vi "WriteTree.vi"(8 "error in":errorcluster, 11 "repository in":refnum<class "NISE_CEF_HierarchyRepo.lvclass">) -> (0 "error out":errorcluster, 2 "root":T1, 3 "repository out":refnum<class "NISE_CEF_Repository.lvclass">)   [LabVIEW 2013, in "NISE_CEF_HierarchyRepo.lvclass"]
doc: "Transfers information between the repo and the tree control. This method should be called after the custom views are called or saving to disk."
uses:
  NISE_CEF_HierarchyRepo.lvclass
  Repository/NISE_CEF_Repository.lvclass
  Node/NodeRef.ctl
  Node/NISE_CEF_Node.lvclass
  Node/FromRepoCluster.ctl
  NISE_CEF_HierarchyRepo.lvclass/NISE_CEF_HierarchyRepo.ctl
  serializable node/NISE_CEF_serializable node.lvclass
  tree based serializer/NISE_CEF_TreeSerializer.lvlib
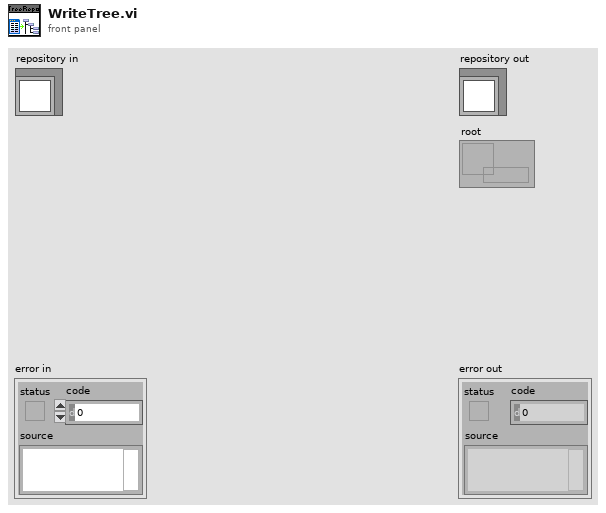
[diagram p1: front panel]
types:
  T1 = typedef "NISE_CEF_Node.lvclass/NodeRef.ctl" = refnum<data-value>
  T2 = typedef "NISE_CEF_Node.lvclass/FromRepoCluster.ctl" = cluster{"tag":string, "tags":string[], "classes":string[], "index":i32, "variant":variant}
  T3 = typedef "NISE_CEF_TreeSerializer.lvlib/memory hierarchy.ctl" = cluster{"root":string, "hierarchy":T4[], "instance data":refnum<class "NISE_CEF_serializable configuration.lvclass">[]}
  T4 = typedef "NISE_CEF_TreeSerializer.lvlib/hierarchy element.ctl" = cluster{"current node":string, "children":string[]}
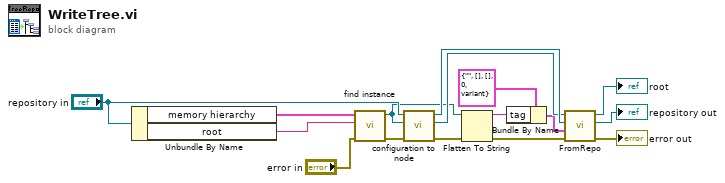
[diagram p0: block diagram]
diagram:
  n1 = Unbundle By Name("repository in") -> ("memory hierarchy"=w11:T3, "root"=w13:string)
  n2 = call "find instance.vi"("error in"="error in", "ID"=w13, "memory hierarchy"=w11) -> ("error out"=w6:errorcluster, "configuration"=w2:refnum<class "NISE_CEF_serializable configuration.lvclass">)  [unwired: 7 in]
  n3 = call-dynamic "configuration to node.vi"("error in"=w6, "configuration"=w2, "hierarchy repo in"="repository in") -> ("error out"=w7:errorcluster, "node"=w8:refnum<class "NISE_CEF_serializable node.lvclass">, "hierarchy repo out"=w9:refnum<class "NISE_CEF_HierarchyRepo.lvclass">)  [unwired: 6 in]
  n4 = Flatten To String(anything=w2, error in (no error)=w7) -> (data string=w1:string, error out=w3:errorcluster)  [unwired: 2 in, 1 out]
  n5 = Bundle By Name(cluster=T2 {"tag"="", "tags"=[], "classes"=[], "index"=0, "variant"=variant} ("from repo cluster"), "tag"=w1) -> (w4:T2)
  n6 = call-dynamic "FromRepo.vi"("error in"=w3, "from repo cluster"=w4, "repository in"=w9, "node in"=w8) -> ("error out"=→"error out":errorcluster, "repository out"=→"repository out":refnum<class "NISE_CEF_Repository.lvclass">, "node"=→"root":T1)  [unwired: 5 in]
